vi "Write pcap format.vi"(8 "error in (no error)":errorcluster, 10 "File Format":T1={"Endian"=enum."Little Endian", "Time Format"=enum."ns"}, 11 "pcap Parse and Build in":refnum<class "pcap Parse and Build.lvclass">) -> (0 "error out":errorcluster, 3 "pcap Parse and Build out":refnum<class "pcap Parse and Build.lvclass">)   [LabVIEW 2021, in "pcap Parse and Build.lvclass"]
uses:
  pcap Parse and Build.lvclass
  Typedef/Time Format.ctl
  <vilib>/CIF Foundation/CIF Utilities/DataTypes/Endian.ctl
  <vilib>/CIF Foundation/CIF Utilities/DataTypes/DataTypes_CIF_U.lvlib
  Typedef/File Format.ctl
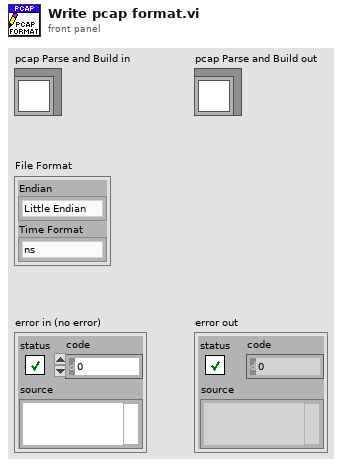
[diagram p1: front panel]
types:
  T1 = typedef "pcap Parse and Build.lvclass/File Format.ctl" = cluster{"Endian":T2, "Time Format":T3}
  T2 = typedef "DataTypes_CIF_U.lvlib/Endian.ctl" = enum16{"Little Endian", "Big Endian"}
  T3 = typedef "pcap Parse and Build.lvclass/Time Format.ctl" = enum16{"us", "ns"}
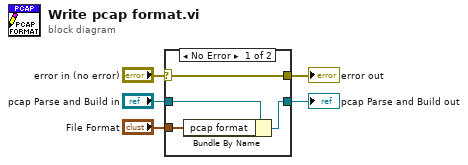
[diagram p0: block diagram]
diagram:
  n1 = case shown="No Error" "error in (no error)" {
    selector: "error in (no error)" -> [w9 w10]
    tunnel: [w9 w10] -> w4
    tunnel: [w7 w11] -> w2
    tunnel: "pcap Parse and Build in" -> [w8 w11]
    tunnel: "File Format" -> [w6 _]
    frame No Error {
      n2 = Bundle By Name(cluster=w8, "pcap format"=w6) -> (w7:refnum<class "pcap Parse and Build.lvclass">)
    }
    frame Error {
    }
  }
  "error out" <- w4
  "pcap Parse and Build out" <- w2
